vi "SetUnits.vi"(8 "error in (no error)":errorcluster, 10 "SystemUnits":T1, 11 "TCP Network Connection in":refnum<k5>) -> (0 "error out":errorcluster, 3 "TCP Network Connection out":refnum<k5>, 5 "Respond":string[](array[string]), 7 "Command":string)   [LabVIEW 2017]
uses:
  AT901 API/Structures/Struct SystemUnits.ctl
  AT901 API/TypeDefinitions/ES_LengthUnit.ctl
  AT901 API/TypeDefinitions/ES_AngleUnit.ctl
  AT901 API/TypeDefinitions/ES_TemperatureUnit.ctl
  AT901 API/TypeDefinitions/ES_PressureUnit.ctl
  AT901 API/TypeDefinitions/ES_HumidityUnit.ctl
  AT901 API/TypeDefinitions/ES_DataType.ctl
  AT901 API/TypeDefinitions/ES_Command.ctl
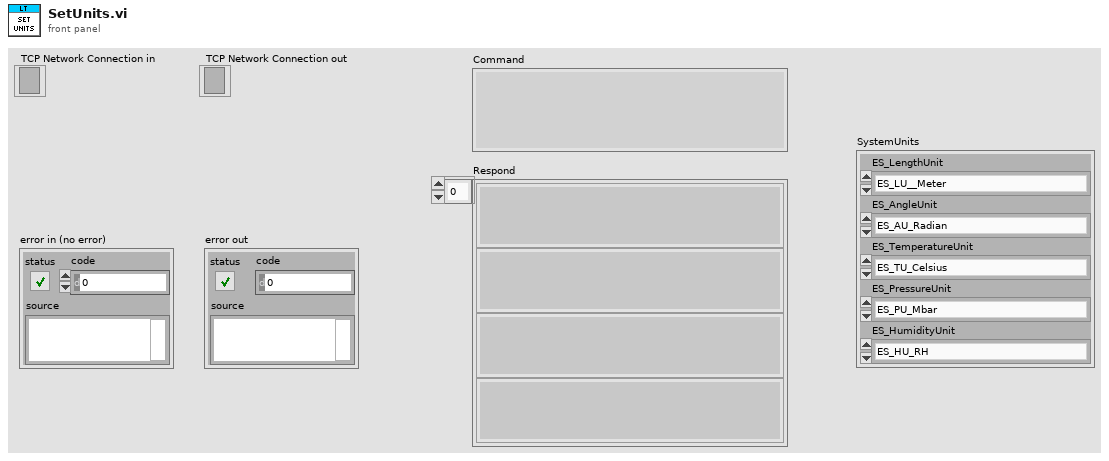
[diagram p1: front panel]
types:
  T1 = typedef "Struct SystemUnits.ctl" = cluster{"ES_LengthUnit":T2, "ES_AngleUnit":T3, "ES_TemperatureUnit":T4, "ES_PressureUnit":T5, "ES_HumidityUnit":T6}
  T2 = typedef "ES_LengthUnit.ctl" = enum32{"ES_LU__Meter", "ES_LU_Millimeter", "ES_LU_Micron", "ES_LU_Foot", "ES_LU_Yard", "ES_LU_Inch"}
  T3 = typedef "ES_AngleUnit.ctl" = enum32{"ES_AU_Radian", "ES_AU_Degree", "ES_AU_Gon"}
  T4 = typedef "ES_TemperatureUnit.ctl" = enum32{"ES_TU_Celsius", "ES_TU_Fahrenheit"}
  T5 = typedef "ES_PressureUnit.ctl" = enum32{"ES_PU_Mbar", "ES_PU_HPascal", "ES_PU_KPascal", "ES_PU_MmHg", "ES_PU_Psi", "ES_PU_InH2O", "ES_PU_InHg"}
  T6 = typedef "ES_HumidityUnit.ctl" = enum32{"ES_HU_RH"}
  T7 = typedef "ES_Command.ctl" = enum32{"ES_C_ExitApplication", "ES_C_GetSystemStatus", "ES_C_GetTrackerStatus", "ES_C_SetTemperatureRange", "ES_C_GetTemperatureRange", "ES_C_SetUnits", "ES_C_GetUnits", "ES_C_Intialize", "ES_C_ReleaseMotors", "ES_C_ActivateCameraView", "ES_C_Park", "ES_C_SwitchLaser", "ES_C_SetStationOriantationParams", "ES_C_GetStationOrientationParams", "ES_C_SetTransformationParams", "ES_C_GetTransformationParams", "ES_C_SetBoxRegionParams", "ES_C_GetBoxRegionParams", "ES_C_SetSphereRegionParams", "ES_C_GetSphereRegionParams", "ES_C_SetEnvironmentParams", "ES_C_GetEnvironmentParams", "ES_C_SetRefractionParams", "ES_C_GetRefractionParams", "ES_C_SetMeasurementMode", "ES_C_GetMeasurementMode", "ES_C_SetCoordinateSystemType", "ES_C_GetCoordinateSystemType", "ES_C_SetStationaryModeParams", "ES_C_GetStationaryModeParams", "ES_C_SetContinuousTimeModeParams", "ES_C_GetContinuousTimeModeParams", "ES_C_SetContinuousDistanceModeParams", "ES_C_GetContinuousDistanceModeParams", "ES_C_SetSphereCenterModeParams", "ES_C_GetSphereCenterModeParams", "ES_C_SetCircleCenterModeParams", "ES_C_GetCircleCenterModeParams", "ES_C_SetGridModeParams", "ES_C_GetGridModeParams", "ES_C_SetReflector", "ES_C_GetReflector", "ES_C_GetReflectors", "ES_C_SetSearchParams", "ES_C_GetSearchParams", "ES_C_SetAdmParams", "ES_C_GetAdmParams", "ES_C_SetSystemSettings", "ES_C_GetSystemSettings", "ES_C_StartMeasurement", "ES_C_Start6DMeasurement", "ES_C_StartNivelMeasurement", "ES_C_StopMeasurement", "ES_C_ChangeFace", "ES_C_GoBirdBath", "ES_C_GoPosition", "ES_C_GoPositionHVD", "ES_C_PositionRelativeHV", "ES_C_PointLaser", "ES_C_PointLaserHVD", "ES_C_MoveHV", "ES_C_GoNivelPosition", "ES_C_GoLastMeasuredPoint", "ES_C_FindReflector", "ES_C_Unknown", "ES_C_LookForTarget", "ES_C_GetDirection", "ES_C_CallOrientToGravity", "ES_C_ClearTransformationNominalPointList", "ES_C_ClearTransformationActualPointList", "ES_C_AddTransformationNominalPoint", "ES_C_AddTransformationActualPoint", "ES_C_SetTransformationInputParams", "ES_C_GetTransformationInputParams", "ES_C_CallTransformation", "ES_C_GetTransformedPoints", "ES_C_ClearDerivePointList", "ES_C_AddDrivePoint", "ES_C_CallIntermediateCompensation", "ES_C_SetCompensation", "ES_C_SetStatisticMode", "ES_C_GetStatisticMode", "ES_C_GetStillImage", "ES_C_SetCameraParams", "ES_C_GetCameraParams", "ES_C_GetCompensation", "ES_C_GetCompensations", "ES_C_CheckBirdBath", "ES_C_GetTrackerDiagnostics", "ES_C_GetADMInfo", "ES_C_GetTPInfo", "ES_C_GetNivelInfo", "ES_C_SetLaserOnTimer", "ES_C_GetLaserOnTimer", "ES_C_ConvertDisplayCoordinates", "ES_C_GorBirdBath2", "ES_C_SetTriggerSource", "ES_C_GetTriggerSource", "ES_C_GetFace", "ES_C_GetCameras", "ES_C_GetCamera", "ES_C_SetMeasurementCameraMode", "ES_C_GetMeasurementCameraMode", "ES_C_GetProbes", "ES_C_GetProbe", "ES_C_GetTipAdapters", "ES_C_GetTipAdapter", "ES_C_GetTCamToTrackerCompensations", "ES_C_GetTCamToTrackerCompensation", "ES_C_SetTCamToTrackerCompensation", "ES_C_GetProbeCompensations", "ES_C_GetProbeCompensation", "ES_C_SetProbeCompensation", "ES_C_GetTipToProbeCompensations", "ES_C_GetTipToProbeCompensation", "ES_C_SetExternTriggerParams", "ES_C_GetExternTriggerParams", "ES_C_GetErrorEllipsoid", "ES_C_GetMeasurementCameraInfo", "ES_C_GetMeasurementProbeInfo", "ES_C_SetLongSystemParameter", "ES_C_GetLongSystemParameter", "ES_C_GetMeasurementStatusInfo", "ES_C_GetCompensations2", "ES_C_GetCurrentPrismPosition", "ES_C_SetDoubleSystemParameter", "ES_C_GetDoubleSystemParameter", "ES_C_GetObjectTemperature", "ES_C_GetTriggerBoardInfo", "ES_C_GetOverviewCameraInfo", "ES_C_ClearCommandQueue", "ES_C_GetADMInfo2", "ES_C_GetTrackerInfo", "ES_C_GetNivelInfo2", "ES_C_RestoreStartupConditions", "ES_C_GoAndMeasure", "ES_C_GetTipToProbeCompensation2", "SetPowerLockMode", "GetPowerLockMode", "SetPowerLockFunctionAvailable", "GetPowerLockFunctionAvailable"}
  T8 = typedef "ES_DataType.ctl" = enum32{"ES_DT_Command", "ES_DT_Error", "ES_DT_SingleMeasResult", "ES_DT_MultiMeasResult", "ES_DT_StationaryProbeMeasResult", "ES_DT_ContinuousProbeMeasResult", "ES_DT_NivelResult", "ES_DT_ReflectorPosResult", "ES_DT_SystemStatusChange", "ES_DT_SingleMeasResult2", "ES_DT_MultiMeasResult2", "ES_DT_ProbePosResult"}
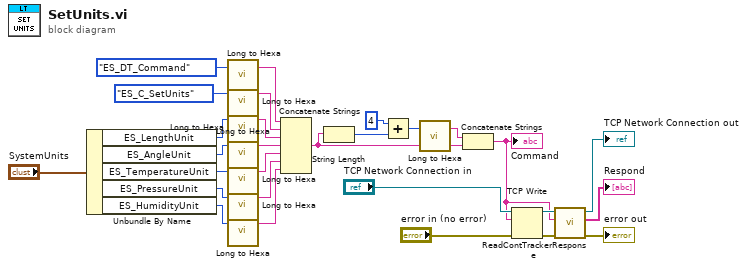
[diagram p0: block diagram]
diagram:
  n1 = Unbundle By Name("SystemUnits") -> ("ES_LengthUnit"=w6:T2, "ES_AngleUnit"=w7:T3, "ES_TemperatureUnit"=w8:T4, "ES_PressureUnit"=w9:T5, "ES_HumidityUnit"=w10:T6)
  n2 = call "Long to Hexa.vi"("Long"=ES_DataType."ES_DT_Command" ("ES_DataType")) -> ("Hexa"=w21:string)  [unwired: 2 in]
  n3 = call "Long to Hexa.vi"("Long"=ES_Command."ES_C_SetUnits" ("ES_Command")) -> ("Hexa"=w22:string)  [unwired: 2 in]
  n4 = call "Long to Hexa.vi"("Long"=w6) -> ("Hexa"=w5:string)  [unwired: 2 in]
  n5 = call "Long to Hexa.vi"("Long"=w7) -> ("Hexa"=w4:string)  [unwired: 2 in]
  n6 = call "Long to Hexa.vi"("Long"=w8) -> ("Hexa"=w3:string)  [unwired: 2 in]
  n7 = call "Long to Hexa.vi"("Long"=w9) -> ("Hexa"=w2:string)  [unwired: 2 in]
  n8 = call "Long to Hexa.vi"("Long"=w10) -> ("Hexa"=w1:string)  [unwired: 2 in]
  n9 = Concatenate Strings(w21, w22, w5, w4, w3, w2, w1) -> (w19:string)
  n10 = String Length(string=w19) -> (length=w16:i32)
  n11 = Add(x=4 ("Index"), y=w16) -> (x+y=w18:i32)
  n12 = call "Long to Hexa.vi"("Long"=w18) -> ("Hexa"=w20:string)  [unwired: 2 in]
  n13 = Concatenate Strings(w20, w19) -> (w12:string)
  "Command" <- w12
  n14 = TCP Write(connection ID="TCP Network Connection in", data in=w12, error in (no error)="error in (no error)") -> (connection ID out=w23:refnum<k5>, error out=w25:errorcluster)  [unwired: 1 in, 1 out]
  n15 = call "ReadContTrackerResponse.vi"("error in (no error)"=w25, "Command"=w12, "TCP Network Connection in"=w23) -> ("error out"=→"error out":errorcluster, "Respond"=→"Respond":string[], "TCP Network Connection out"=→"TCP Network Connection out":refnum<k5>)  [unwired: 6 in]
